vi "Load Settings from JSON.vi"(8 "error in (no error)":errorcluster, 11 "JSON String":string) -> (0 "error out":errorcluster, 3 "Settings out":T1={"Plug-in Version"="", "Step Values"=[], "Only Execute When Test Running"=TRUE, "Reset Sequence When Test Starts"=TRUE, "Number of Sequence Steps"=0, "Num of Analog Channels"=0, "Num of Digital Channels"=0, "Delay Before Starting Sequence"=0.0, "Default Analog Values"=[], "Default Digital Values"=[], "Max Iterations"=0, "Use last value when stopped"=FALSE, "Prioritize exact values"=FALSE, "Enable advanced step timing"=FALSE, "Enable step conditions"=FALSE, "Show confirmation dialogs"=FALSE, "Start condition"="", "Enable re-triggering"=FALSE, "Stop condition"=""})   [LabVIEW 2020, in "Output Sequencer.lvlib" / "Output Sequencer.lvclass"]
uses:
  Output Sequencer.lvclass
  Output Sequencer.lvclass/Output Sequencer.ctl
  494bb6af-513b-4fa7-a84a-c35cc4f9ba6f.vi
  Globals/Global Strings.vi
  Settings UI/Types/Step Settings.ctl
  Settings UI/Settings UI.lvclass
  Settings UI/Types/Settings.ctl
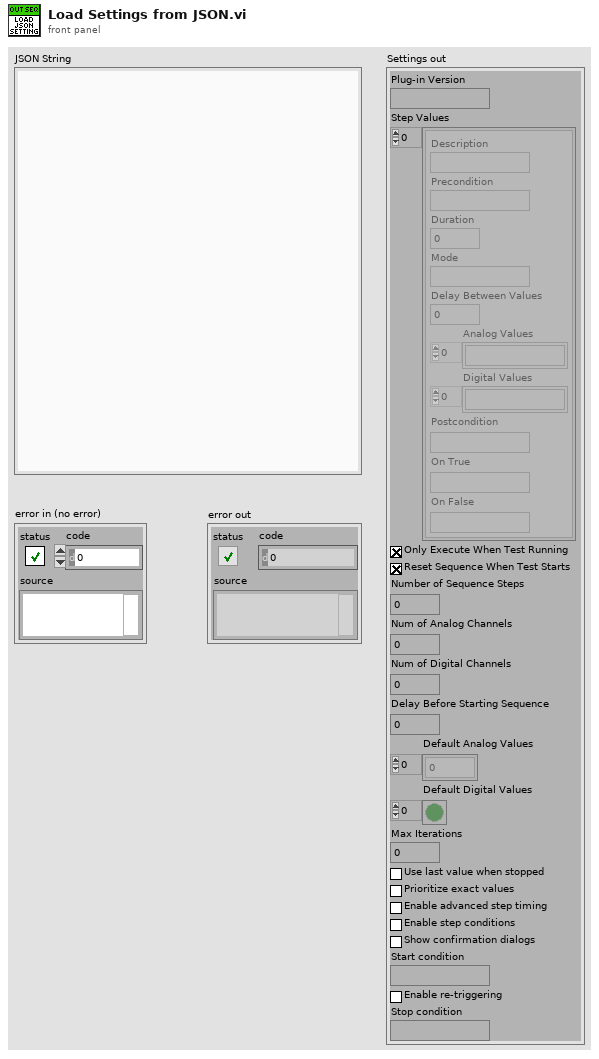
[diagram p1: front panel]
types:
  T1 = typedef "Output Sequencer.lvlib/Settings UI.lvclass/Settings.ctl" = cluster{"Plug-in Version":string, "Step Values":T2[], "Only Execute When Test Running":bool, "Reset Sequence When Test Starts":bool, "Number of Sequence Steps":i32, "Num of Analog Channels":i32, "Num of Digital Channels":i32, "Delay Before Starting Sequence":dbl, "Default Analog Values":dbl[], "Default Digital Values":bool[], "Max Iterations":u32, "Use last value when stopped":bool, "Prioritize exact values":bool, "Enable advanced step timing":bool, "Enable step conditions":bool, "Show confirmation dialogs":bool, "Start condition":string, "Enable re-triggering":bool, "Stop condition":string}
  T2 = typedef "Output Sequencer.lvlib/Settings UI.lvclass/Step Settings.ctl" = cluster{"Description":string, "Precondition":string, "Duration":dbl, "Mode":string, "Delay Between Values":dbl, "Analog Values":string[], "Digital Values":string[], "Postcondition":string, "On True":string, "On False":string}
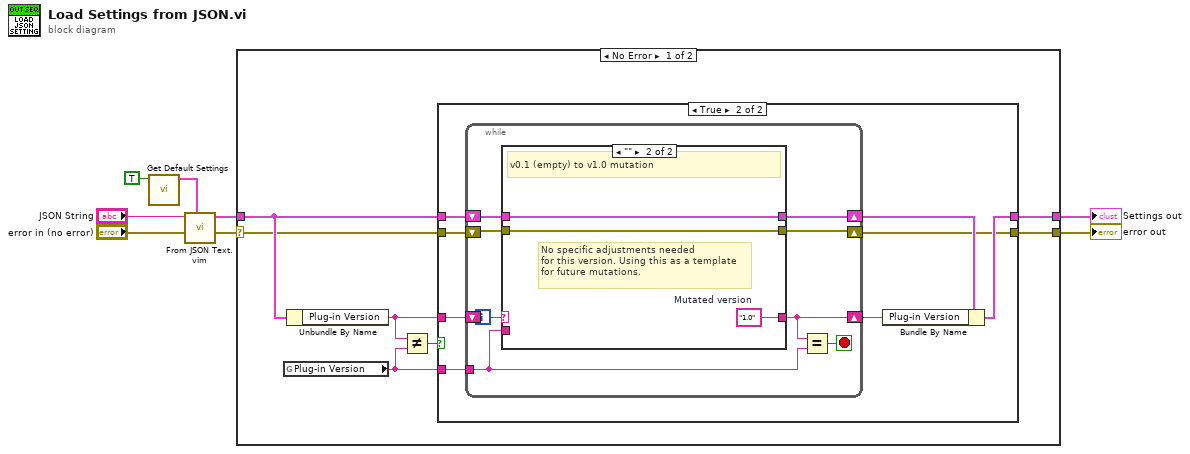
[diagram p0: block diagram]
diagram:
  n1 = call "Get Default Settings.vi"("For Load (F)"=TRUE) -> ("Settings out"=w2:T1)  [unwired: 9 in, 1 out]
  n2 = call "From JSON Text.vim"("Data Type and Default Value"=w2, "error in (no error)"="error in (no error)", "JSON"="JSON String") -> ("error out"=w4:errorcluster, "Data out"=w6:T1)  [unwired: 7 in]
  n3 = case shown="No Error" w4 {
    selector: w4 -> [w11 w41]
    tunnel: [w9 w40] -> w8
    tunnel: w6 -> [w14 w40]
    tunnel: [w10 w41] -> w3
    frame No Error {
      n4 = global read "Global Strings.vi" "Plug-in Version"() -> (w13:string)
      n5 = Unbundle By Name(w14) -> ("Plug-in Version"=w12:string)
      n6 = Not Equal?(x=w12, y=w13) -> (x != y?=w15:bool)
      n7 = case shown="True" w15 {
        tunnel: w14 -> [w17 w22]
        tunnel: w13 -> [_ w23]
        tunnel: [w17 w25] -> w9
        tunnel: w12 -> [_ w24]
        tunnel: w11 -> [w16 w19]
        tunnel: [w16 w18] -> w10
        frame False {
        }
        frame True {
          n8 = while {
            shift-right: [w31] -> w20
            shift-left: w24 -> [w33]
            tunnel: w23 -> [w28]
            shift-right: [w27] -> w18
            shift-left: w19 -> [w26]
            shift-right: [w29] -> w21
            shift-left: w22 -> [w30]
            stop <- w32 stop-if-true
            n9 = case shown="\"\"" w33 {
              tunnel: [w35 w39] -> w31
              tunnel: w30 -> [w36 w38]
              tunnel: [w36 w38] -> w29
              tunnel: w28 -> [w35 _]
              tunnel: [w34 w37] -> w27
              tunnel: w26 -> [w34 w37]
              frame Default {
                # "Set mutated version to current version"
                # "No mutation specified. Assume no \nadditional mutations required for this version."
              }
              frame "" {
                w39 = "1.0"  # Mutated version
                # "No specific adjustments needed\nfor this version. Using this as a template\nfor future mutations."
                # "v0.1 (empty) to v1.0 mutation"
              }
            }
            n10 = Equal?(x=w31, y=w28) -> (x = y?=w32:bool)
          }
          n11 = Bundle By Name(cluster=w21, "Plug-in Version"=w20) -> (w25:T1)
        }
      }
    }
    frame Error {
    }
  }
  "Settings out" <- w8
  "error out" <- w3
